vi "Initialize.vi"(2 "XRef":refnum<vi>) -> (1 "State Out":T1={"Input Type"=variant(dbl 0.0), "Selection"=0, "Element Names"=[], "Type Strings"=[], "Element Types"=[]})   [LabVIEW 2015, in "Construct-Tagged-Union.xnode"]
doc: "This ability VI is called when your XNode is first dropped. It is used to specify your initial state.\n\nDefault behavior: Intialize state to default defaults (usually zero-initialized).\n\nThis ability does not provide UI and OS messages are not handled.\n\nSee also: Copy"
uses:
  Construct-Tagged-Union.xnode
  State.ctl
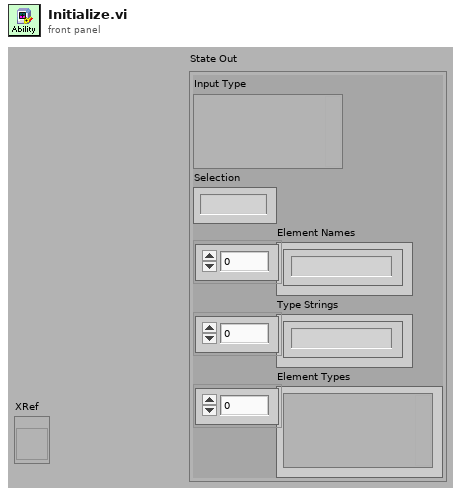
[diagram p1: front panel]
types:
  T1 = typedef "Construct-Tagged-Union.xnode/State.ctl" = cluster{"Input Type":variant, "Selection":i32, "Element Names":string[], "Type Strings":string[], "Element Types":variant[]}
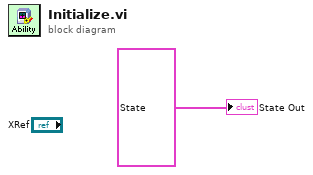
[diagram p0: block diagram]
diagram:
  "State Out" <- T1 {"Input Type"=variant, "Selection"=0, "Element Names"=[], "Type Strings"=[], "Element Types"=[]} ("State")
